vi "Handle Anomaly Log.vi"(0 "Data":dbl[][](array[numeric]), 5 "Enable":bool, 7 "RowCount In":i32, 9 "Anomaly Log Path":path, 11 "Current Data Path":path) -> ()   [LabVIEW 2013]
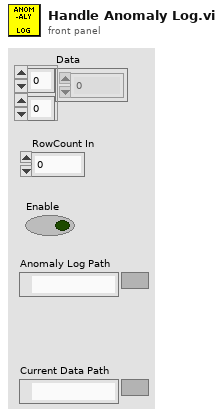
[diagram p1: front panel]
types:
  T1 = enum16{"open", "replace", "create", "open or create", "replace or create", "replace or create with confirmation"}
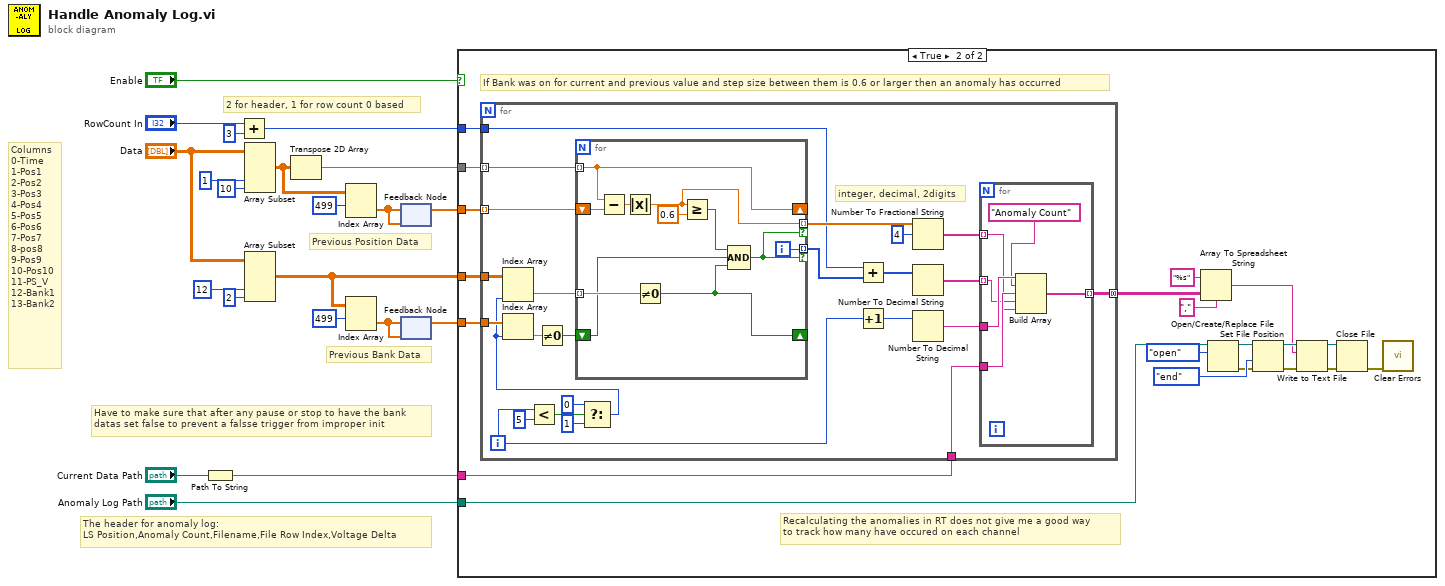
[diagram p0: block diagram]
diagram:
  # "Have to make sure that after any pause or stop to have the bank\ndatas set false to prevent a falsse trigger from improper init"
  # "Previous Position Data"
  # "Previous Bank Data"
  # "2 for header, 1 for row count 0 based"
  # "The header for anomaly log:\nLS Position,Anomaly Count,Filename,File Row Index,Voltage Delta"
  # "Columns\n0-Time\n1-Pos1\n2-Pos2\n3-Pos3\n4-Pos4\n5-Pos5\n6-Pos6\n7-Pos7\n8-pos8\n9-Pos9\n10-Pos10\n11-PS_V\n12-Bank1\n13-Bank2"
  n1 = Path To String(path="Current Data Path") -> (string=w13:string)
  n2 = Add(x="RowCount In", y=3 ("x")) -> (x+y=w15:i32)
  n3 = Array Subset(array="Data", index (col)=1 ("index"), length (col)=10 ("length")) -> (w3:dbl[][])  [unwired: 2 in]
  n4 = Array Subset(array="Data", index (col)=12 ("index"), length (col)=2 ("length")) -> (w9:dbl[][])  [unwired: 2 in]
  n5 = Transpose 2D Array(2D array=w3) -> (transposed array=w16:dbl[][])
  n6 = Index Array(array=w3, index (row)=499) -> (element=w5:dbl[])  [unwired: 1 in]
  n7 = Index Array(array=w9, index (row)=499) -> (element=w7:dbl[])  [unwired: 1 in]
  n8 = feedback #1(w5) -> (w2:dbl[])
  n9 = feedback-in #1(w5) -> ()
  n10 = feedback-in #2(w7) -> ()
  n11 = feedback #2(w7) -> (w6:dbl[])
  n12 = case shown="True" "Enable" {
    tunnel: w16 -> [_ w41]
    tunnel: w15 -> [_ w40]
    tunnel: w13 -> [_ w39]
    tunnel: "Anomaly Log Path" -> [_ w25]
    tunnel: w9 -> [_ w24]
    tunnel: w6 -> [_ w23]
    tunnel: w2 -> [_ w22]
    frame False {
    }
    frame True {
      # "Recalculating the anomalies in RT does not give me a good way\nto track how many have occured on each channel"
      # "If Bank was on for current and previous value and step size between them is 0.6 or larger then an anomaly has occurred"
      n13 = for {
        tunnel: w41 -> [w56] mode=indexing
        tunnel: w24 -> [w61]
        tunnel: w22 -> [w57] mode=indexing
        tunnel: w23 -> [w60]
        tunnel: w40 -> [w50]
        tunnel: w39 -> [w43]
        tunnel: [w42] -> w27 mode=concatenating
        i -> [w51]
        # "integer, decimal, 2digits"
        n14 = Less?(x=w51, y=5) -> (x < y?=w64:bool)
        n15 = Select(t=0 ("index"), s=w64, f=1 ("index")) -> (s? t:f=w59:i32)
        n16 = Index Array(array=w61, index (col)=w59) -> (element=w58:dbl[])  [unwired: 1 in]
        n17 = Index Array(array=w60, index=w59) -> (element=w55:dbl)
        n18 = Not Equal To 0?(x=w55) -> (x != 0?=w54:bool)
        n19 = for {
          tunnel: w56 -> [w81] mode=indexing
          tunnel: w58 -> [w82] mode=indexing
          shift-right: [w81] -> _
          shift-left: w57 -> [w80]
          shift-right: [w75] -> _
          shift-left: w54 -> [w76]
          tunnel: [w74] -> w49 mode=indexing if=w72
          tunnel: [w73] -> w53 mode=indexing if=w72
          i -> [w74]
          n20 = Subtract(x=w81, y=w80) -> (x-y=w79:dbl)
          n21 = Absolute Value(x=w79) -> (abs(x)=w73:dbl)
          n22 = Not Equal To 0?(x=w82) -> (x != 0?=w75:bool)
          n23 = Greater Or Equal?(x=w73, y=0.6) -> (x >= y?=w77:bool)
          n24 = Compound Arithmetic op=AND(w77, w76, w75) -> (w72:bool)
        }
        n25 = Add(x=w50, y=w49) -> (x+y=w48:i32[])
        n26 = Increment(x=w51) -> (x+1=w47:i32)
        n27 = Number To Fractional String(number=w53, width (-)=i16 4) -> (F-format string=w46:string[])  [unwired: 2 in]
        n28 = Number To Decimal String(number=w48) -> (decimal integer string=w45:string[])  [unwired: 1 in]
        n29 = Number To Decimal String(number=w47) -> (decimal integer string=w44:string)  [unwired: 1 in]
        n30 = for {
          tunnel: w46 -> [w67] mode=indexing
          tunnel: w45 -> [w68] mode=indexing
          tunnel: w44 -> [w71]
          tunnel: w43 -> [w69]
          tunnel: [w66] -> w42 mode=indexing
          n31 = Build Array(w71, "Anomaly Count" ("element"), w69, w68, w67) -> (w66:string[])
        }
      }
      n32 = Array To Spreadsheet String(delimiter (Tab)=",", array=w27, 3:"%s" ("format string")) -> (spreadsheet string=w26:string)
      n33 = Open/Create/Replace File(file path (use dialog)=w25, operation (0:open)=T1."open") -> (refnum out=w34:refnum<file>, error out=w35:errorcluster)  [unwired: 4 in, 1 out]
      n34 = Set File Position(refnum=w34, from (0:start)=enum16{"start", "end", "current"}."end", error in=w35) -> (refnum out=w37:refnum<file>, error out=w38:errorcluster)  [unwired: 1 in]
      n35 = Write to Text File(file (use dialog)=w37, text=w26, error in=w38) -> (refnum out=w31:refnum<file>, error out=w30:errorcluster)  [unwired: 1 in, 1 out]
      n36 = Close File(refnum=w31, error in=w30) -> (error out=w32:errorcluster)  [unwired: 1 out]
      n37 = call <vilib>:"Clear Errors.vi"("error in (no error)"=w32) -> ()  [unwired: 6 in, 1 out]
    }
  }
